vi "__ValidateDataTD.vi"(6 "Exactly Match?(F)":bool, 7 "Expected Data":variant, 8 "error in (no error)":errorcluster, 10 "name(\"\" as default, use data name)":string, 11 "Data":variant) -> (0 "error out":errorcluster, 3 "Data out":variant)   [LabVIEW 2019]
uses:
  <userlib>/NEVSTOP-Programming-Palette/Configuration/ClusterCfgTable/ClusterCfgTable_nevstop.lvlib
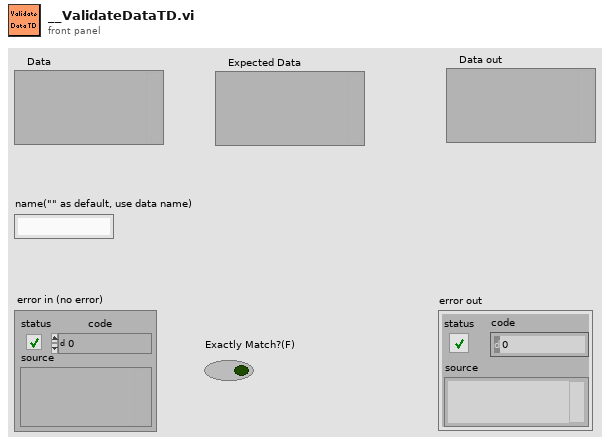
[diagram p1: front panel]
types:
  T1 = typedef "Type Descriptor Enumeration__ogtk.ctl" = enum8{"<Null>", "I8", "I16", "I32", "I64", "U8", "U16", "U32", "U64", "SGL", "DBL", "EXT", "CSG", "CDB", "CXT", "0x0F", "0x10", "0x11", "0x12", "0x13", "0x14", "Enum U8", "Enum U16", "Enum U32", "Enum U64", "SGL PQ", "DBL PQ", "EXT PQ", "CSG PQ", "CDB PQ", "CXT PQ", "0x1F", "0x20", "Boolean", "0x22", "0x23", "0x24", "0x25", "0x26", "0x27", "0x28", "0x29", "0x2A", "0x2B", "0x2C", "0x2D", "0x2E", "0x2F", "String", "0x31", "Path", "Pict", "0x34", "0x35", "0x36", "DAQ", "0x38", "0x39", "0x3A", "0x3B", "0x3C", "0x3D", "0x3E", "0x3F", "Array", "0x41", "0x42", "0x43", "0x44", "0x45", "0x46", "0x47", "0x48", "0x49", "0x4A", "0x4B", "0x4C", "0x4D", "0x4E", "0x4F", "Cluster", "0x51", "0x52", "Variant", "Waveform", "0x55", "0x56", "0x57", "0x58", "0x59", "0x5A", "0x5B", "0x5C", "0x5D", "0x5E", "0x5F", "0x60", "0x61", "0x62", "0x63", "0x64", "0x65", "0x66", "0x67", "0x68", "0x69", "0x6A", "0x6B", "0x6C", "0x6D", "0x6E", "0x6F", "Refnum"}
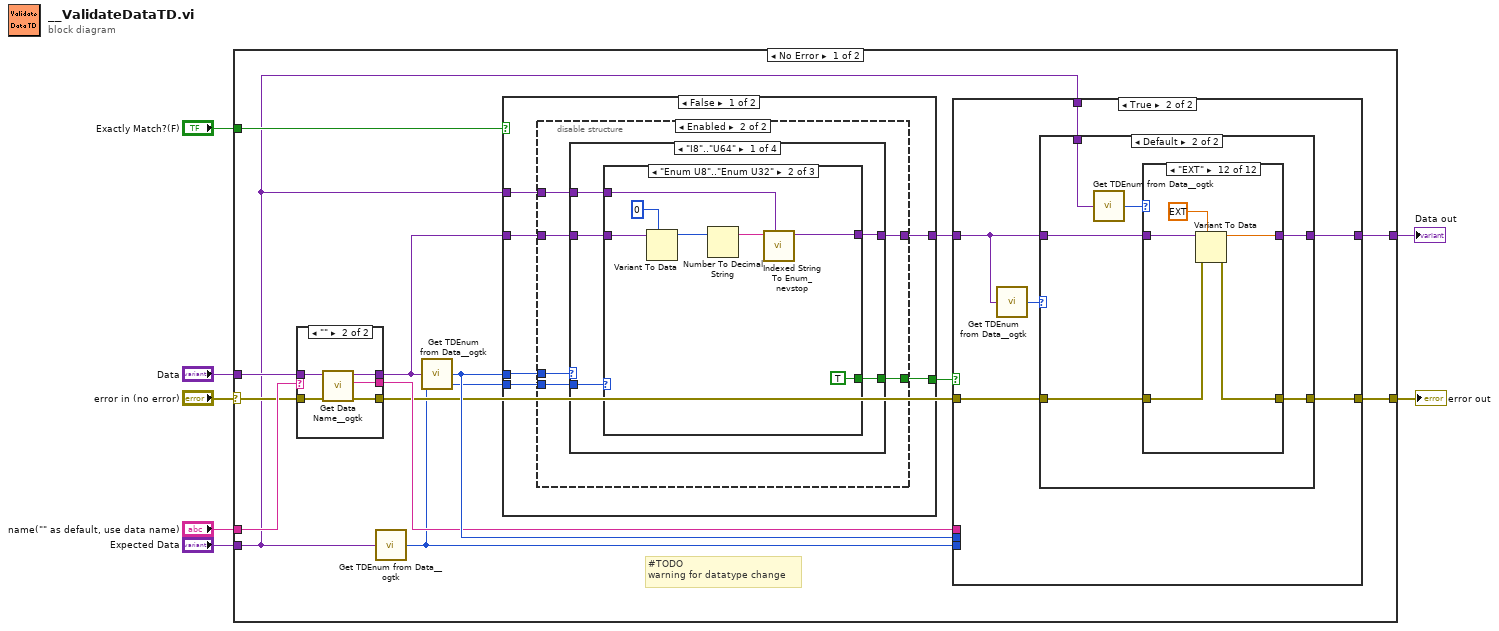
[diagram p0: block diagram]
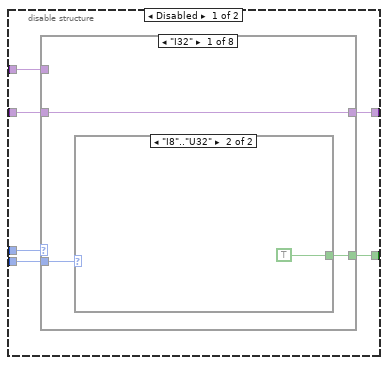
[diagram p2: hidden frame]
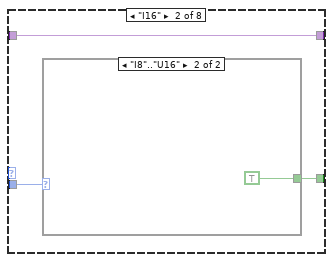
[diagram p4: hidden frame]
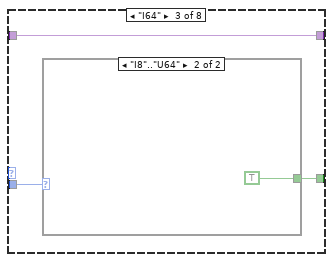
[diagram p6: hidden frame]
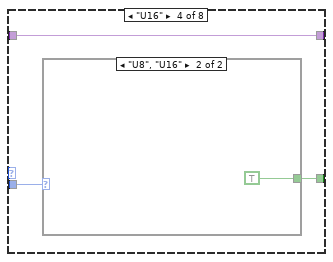
[diagram p8: hidden frame]
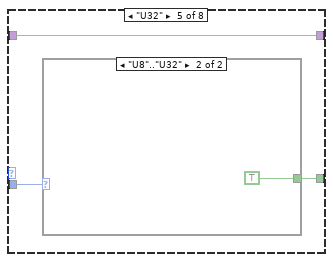
[diagram p10: hidden frame]
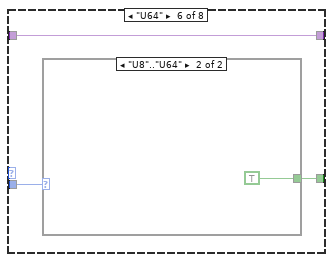
[diagram p12: hidden frame]
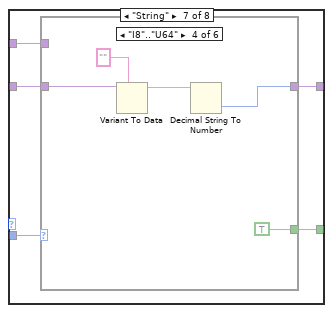
[diagram p14: hidden frame]
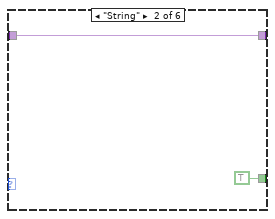
[diagram p16: hidden frame]
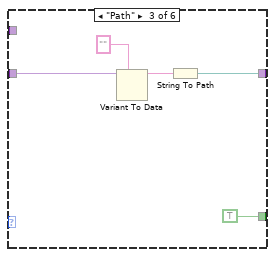
[diagram p17: hidden frame]
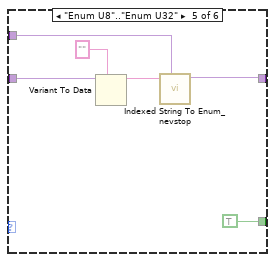
[diagram p18: hidden frame]
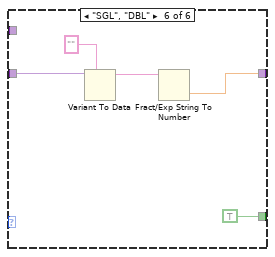
[diagram p19: hidden frame]
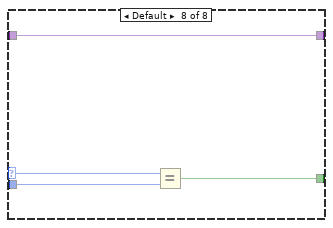
[diagram p20: hidden frame]
diagram:
  n1 = case shown="No Error" "error in (no error)" {
    selector: "error in (no error)" -> [w16 w243]
    tunnel: "Data" -> [w19 w242]
    tunnel: "name(\"\" as default, use data name)" -> [w17 _]
    tunnel: [w18 w243] -> w4
    tunnel: "Expected Data" -> [w8 _]
    tunnel: "Exactly Match?(F)" -> [w13 _]
    tunnel: [w9 w242] -> w1
    frame No Error {
      # "#TODO\nwarning for datatype change"
      n2 = case shown="\"\"" w17 {
        selector: w17 -> [w153 _]
        tunnel: w19 -> [w155 w160]
        tunnel: [w155 w159] -> w12
        tunnel: w16 -> [w154 w158]
        tunnel: [w154 w157] -> w14
        tunnel: [w153 w156] -> w15
        frame Default {
        }
        frame "" {
          n3 = call <userlib>:"Get Data Name__ogtk.vi"("error in (no error)"=w158, "Data"=w160) -> ("error out"=w157:errorcluster, "Data Name"=w156:string, "Data dup"=w159:variant)  [unwired: 7 in]
        }
      }
      n4 = call <userlib>:"Get TDEnum from Data__ogtk.vi"("Data"=w8) -> ("Type Descriptor Enumeration"=w11:T1)  [unwired: 4 in]
      n5 = call <userlib>:"Get TDEnum from Data__ogtk.vi"("Data"=w12) -> ("Type Descriptor Enumeration"=w20:T1)  [unwired: 4 in]
      n6 = case shown="False" w13 {
        tunnel: [w25 w152] -> w21
        tunnel: w20 -> [w27 w151]
        tunnel: w11 -> [w26 w150]
        tunnel: w12 -> [w23 w149]
        tunnel: [w24 w149] -> w10
        tunnel: w8 -> [w22 _]
        frame False {
          n7 = disable-structure shown="Enabled" {
            disable-tunnel: w27 -> [w33 w96]
            disable-tunnel: w26 -> [w32 w95]
            disable-tunnel: [w31 w94] -> w25
            disable-tunnel: [w30 w93] -> w24
            disable-tunnel: w23 -> [w29 w92]
            disable-tunnel: w22 -> [w28 w91]
            frame Disabled {
              n8 = case shown="\"I32\"" w33 {
                selector: w33 -> [_ _ _ _ _ _ _ w90]
                tunnel: w32 -> [w36 w40 w44 w48 w52 w56 w62 w89]
                tunnel: [w35 w39 w43 w47 w51 w55 w59 w88] -> w31
                tunnel: [w34 w38 w42 w46 w50 w54 w61 w87] -> w30
                tunnel: w29 -> [w34 w38 w42 w46 w50 w54 w60 w87]
                tunnel: w28 -> [_ _ _ _ _ _ w58 _]
                frame "I32" {
                  n9 = case shown="\"I8\"..\"U32\"" w36 {
                    tunnel: [_ TRUE] -> w35
                    frame "<Null>", Default {
                    }
                    frame "I8".."U32" {
                    }
                  }
                }
                frame "I16" {
                  n10 = case shown="\"I8\"..\"U16\"" w40 {
                    tunnel: [_ TRUE] -> w39
                    frame "<Null>", Default {
                    }
                    frame "I8".."U16" {
                    }
                  }
                }
                frame "I64" {
                  n11 = case shown="\"I8\"..\"U64\"" w44 {
                    tunnel: [_ TRUE] -> w43
                    frame "<Null>", Default {
                    }
                    frame "I8".."U64" {
                    }
                  }
                }
                frame "U16" {
                  n12 = case shown="\"U8\", \"U16\"" w48 {
                    tunnel: [_ TRUE] -> w47
                    frame "<Null>", Default {
                    }
                    frame "U8", "U16" {
                    }
                  }
                }
                frame "U32" {
                  n13 = case shown="\"U8\"..\"U32\"" w52 {
                    tunnel: [_ TRUE] -> w51
                    frame "<Null>", Default {
                    }
                    frame "U8".."U32" {
                    }
                  }
                }
                frame "U64" {
                  n14 = case shown="\"U8\"..\"U64\"" w56 {
                    tunnel: [_ TRUE] -> w55
                    frame "<Null>", Default {
                    }
                    frame "U8".."U64" {
                    }
                  }
                }
                frame "String" {
                  n15 = case shown="\"I8\"..\"U64\"" w62 {
                    tunnel: [w63 w65 w68 w71 w77 w82] -> w61
                    tunnel: w60 -> [w63 w65 w70 w75 w81 w86]
                    tunnel: [_ TRUE TRUE TRUE TRUE TRUE] -> w59
                    tunnel: w58 -> [_ _ _ _ w76 _]
                    frame "<Null>", Default {
                    }
                    frame "String" {
                    }
                    frame "Path" {
                      n16 = Variant To Data(type="", Variant=w70) -> (data=w69:string)  [unwired: 1 in, 1 out]
                      n17 = String To Path(string=w69) -> (path=w68:path)
                    }
                    frame "I8".."U64" {
                      n18 = Variant To Data(type="", Variant=w75) -> (data=w72:string)  [unwired: 1 in, 1 out]
                      n19 = Decimal String To Number(string=w72) -> (number=w71:i32)  [unwired: 2 in, 1 out]
                    }
                    frame "Enum U8".."Enum U32" {
                      n20 = Variant To Data(type="", Variant=w81) -> (data=w78:string)  [unwired: 1 in, 1 out]
                      n21 = call <userlib>:"Indexed String To Enum_nevstop.vi"("Variant"=w76, "String"=w78) -> ("Enum"=w77:variant)  [unwired: 8 in, 1 out]
                    }
                    frame "SGL", "DBL" {
                      n22 = Variant To Data(type="", Variant=w86) -> (data=w83:string)  [unwired: 1 in, 1 out]
                      n23 = Fract/Exp String To Number(string=w83) -> (number=w82:dbl)  [unwired: 3 in, 1 out]
                    }
                  }
                }
                frame Default {
                  n24 = Equal?(x=w90, y=w89) -> (x = y?=w88:bool)
                }
              }
            }
            frame Enabled {
              n25 = case shown="\"I8\"..\"U64\"" w96 {
                selector: w96 -> [_ _ _ w148]
                tunnel: w95 -> [w101 w114 w120 w147]
                tunnel: [w100 w113 w117 w146] -> w94
                tunnel: [w97 w112 w119 w145] -> w93
                tunnel: w92 -> [w98 w112 w118 w145]
                tunnel: w91 -> [w99 _ w116 _]
                frame "I8".."U64" {
                  n26 = case shown="\"Enum U8\"..\"Enum U32\"" w101 {
                    tunnel: [_ TRUE TRUE] -> w100
                    tunnel: w99 -> [_ w109 _]
                    tunnel: w98 -> [w102 w108 w110]
                    tunnel: [w102 w104 w110] -> w97
                    frame "<Null>", Default {
                    }
                    frame "Enum U8".."Enum U32" {
                      n27 = Variant To Data(type=i64 0 ("code"), Variant=w108) -> (data=w106:i64)  [unwired: 1 in, 1 out]
                      n28 = Number To Decimal String(number=w106) -> (decimal integer string=w105:string)  [unwired: 1 in]
                      n29 = call <userlib>:"Indexed String To Enum_nevstop.vi"("Variant"=w109, "String"=w105) -> ("Enum"=w104:variant)  [unwired: 8 in, 1 out]
                    }
                    frame "I8".."U64" {
                    }
                  }
                }
                frame "SGL".."EXT" {
                  n30 = case shown="\"SGL\"..\"EXT\"" w114 {
                    tunnel: [_ TRUE] -> w113
                    frame "<Null>", Default {
                    }
                    frame "SGL".."EXT" {
                    }
                  }
                }
                frame "String" {
                  n31 = case shown="\"Path\"" w120 {
                    tunnel: [w121 w123 w126 w129 w135 w140] -> w119
                    tunnel: w118 -> [w121 w123 w128 w133 w139 w144]
                    tunnel: [_ TRUE TRUE TRUE TRUE TRUE] -> w117
                    tunnel: w116 -> [_ _ _ _ w134 _]
                    frame "<Null>", Default {
                    }
                    frame "String" {
                    }
                    frame "Path" {
                      n32 = Variant To Data(type="", Variant=w128) -> (data=w127:string)  [unwired: 1 in, 1 out]
                      n33 = String To Path(string=w127) -> (path=w126:path)
                    }
                    frame "I8".."U64" {
                      n34 = Variant To Data(type="", Variant=w133) -> (data=w130:string)  [unwired: 1 in, 1 out]
                      n35 = Decimal String To Number(string=w130) -> (number=w129:i32)  [unwired: 2 in, 1 out]
                    }
                    frame "Enum U8".."Enum U32" {
                      n36 = Variant To Data(type="", Variant=w139) -> (data=w136:string)  [unwired: 1 in, 1 out]
                      n37 = call <userlib>:"Indexed String To Enum_nevstop.vi"("Variant"=w134, "String"=w136) -> ("Enum"=w135:variant)  [unwired: 8 in, 1 out]
                    }
                    frame "SGL", "DBL" {
                      n38 = Variant To Data(type="", Variant=w144) -> (data=w141:string)  [unwired: 1 in, 1 out]
                      n39 = Fract/Exp String To Number(string=w141) -> (number=w140:dbl)  [unwired: 3 in, 1 out]
                    }
                  }
                }
                frame Default {
                  n40 = Equal?(x=w148, y=w147) -> (x = y?=w146:bool)
                }
              }
            }
          }
        }
        frame True {
          n41 = Equal?(x=w151, y=w150) -> (x = y?=w152:bool)
        }
      }
      n42 = case shown="True" w21 {
        tunnel: w15 -> [w167 _]
        tunnel: [w169 w175] -> w18
        tunnel: w20 -> [w164 _]
        tunnel: w11 -> [w163 _]
        tunnel: w14 -> [w162 w176]
        tunnel: w10 -> [w161 w172]
        tunnel: [w161 w173] -> w9
        tunnel: w8 -> [_ w174]
        frame False {
          n43 = Format Into String(format string="\"%s\": DataType Not Expected!\n\"%s\" -> Expected: \"%s\"" ("String to Prepend to source (\"\")"), w167, w164, w163) -> (resulting string=w165:string)  [unwired: 2 in, 1 out]
          n44 = call <userlib>:"Build Error Cluster__ogtk.vi"("String to Prepend to source (\"\")"=w165, "code"=1) -> ("error out"=w168:errorcluster)
          n45 = Merge Errors(w162, w168) -> (w169:errorcluster)
        }
        frame True {
          n46 = call <userlib>:"Get TDEnum from Data__ogtk.vi"("Data"=w172) -> ("Type Descriptor Enumeration"=w171:T1)  [unwired: 4 in]
          n47 = case shown="Default" w171 {
            tunnel: w176 -> [w177 w184]
            tunnel: [w177 w183] -> w175
            tunnel: w174 -> [_ w180]
            tunnel: [w178 w182] -> w173
            tunnel: w172 -> [w178 w181]
            frame "<Null>" {
            }
            frame Default {
              n48 = call <userlib>:"Get TDEnum from Data__ogtk.vi"("Data"=w180) -> ("Type Descriptor Enumeration"=w179:T1)  [unwired: 4 in]
              n49 = case shown="\"EXT\"" w179 {
                tunnel: w184 -> [w185 w191 w196 w201 w206 w211 w216 w221 w226 w231 w236 w241]
                tunnel: [w185 w190 w195 w200 w205 w210 w215 w220 w225 w230 w235 w240] -> w183
                tunnel: [w186 w189 w194 w199 w204 w209 w214 w219 w224 w229 w234 w239] -> w182
                tunnel: w181 -> [w186 w188 w193 w198 w203 w208 w213 w218 w223 w228 w233 w238]
                frame "<Null>", Default {
                }
                frame "I8" {
                  n50 = Variant To Data(error in=w191, type=i8 0 ("code"), Variant=w188) -> (data=w189:i8, error out=w190:errorcluster)
                }
                frame "I16" {
                  n51 = Variant To Data(error in=w196, type=i16 0 ("code"), Variant=w193) -> (data=w194:i16, error out=w195:errorcluster)
                }
                frame "I32" {
                  n52 = Variant To Data(error in=w201, type=0 ("code"), Variant=w198) -> (data=w199:i32, error out=w200:errorcluster)
                }
                frame "I64" {
                  n53 = Variant To Data(error in=w206, type=i64 0 ("code"), Variant=w203) -> (data=w204:i64, error out=w205:errorcluster)
                }
                frame "U8" {
                  n54 = Variant To Data(error in=w211, type=u8 0 ("code"), Variant=w208) -> (data=w209:u8, error out=w210:errorcluster)
                }
                frame "U16" {
                  n55 = Variant To Data(error in=w216, type=u16 0 ("code"), Variant=w213) -> (data=w214:u16, error out=w215:errorcluster)
                }
                frame "U32" {
                  n56 = Variant To Data(error in=w221, type=u32 0 ("code"), Variant=w218) -> (data=w219:u32, error out=w220:errorcluster)
                }
                frame "U64" {
                  n57 = Variant To Data(error in=w226, type=u64 0 ("code"), Variant=w223) -> (data=w224:u64, error out=w225:errorcluster)
                }
                frame "SGL" {
                  n58 = Variant To Data(error in=w231, type=sgl 0.0 ("code"), Variant=w228) -> (data=w229:sgl, error out=w230:errorcluster)
                }
                frame "DBL" {
                  n59 = Variant To Data(error in=w236, type=0.0 ("code"), Variant=w233) -> (data=w234:dbl, error out=w235:errorcluster)
                }
                frame "EXT" {
                  n60 = Variant To Data(error in=w241, type=ext 0.0 ("code"), Variant=w238) -> (data=w239:ext, error out=w240:errorcluster)
                }
              }
            }
          }
        }
      }
    }
    frame Error {
    }
  }
  "error out" <- w4
  "Data out" <- w1
